vi "Update.vi"(10 "测试版？":bool, 11 "服务器信息":T1={"host"="27.154.58.30", "port"=8020, "user"="std", "password"="std23506", "远端地址"="/微站/室外总磷总氮高压过滤无主板新电路板/一体化微型水质监测站.exe"}) -> ()   [LabVIEW 2016, in "数据传输系统-03.lvlib" / "update.lvlib"]
uses:
  update.lvlib
  <vilib>/Utility/miscctls.llb/LVPointTypeDef.ctl
panel:
  out "引用输出":refnum<vi>
  out "已下载大小":sgl format="%.2f MB"
  out "滑动杆":dbl(slide) scale=0.0..100.0
  in  "取消按钮":bool
  out "last status string":string caption="最近状态字符串"
  out "command":string caption="命令"
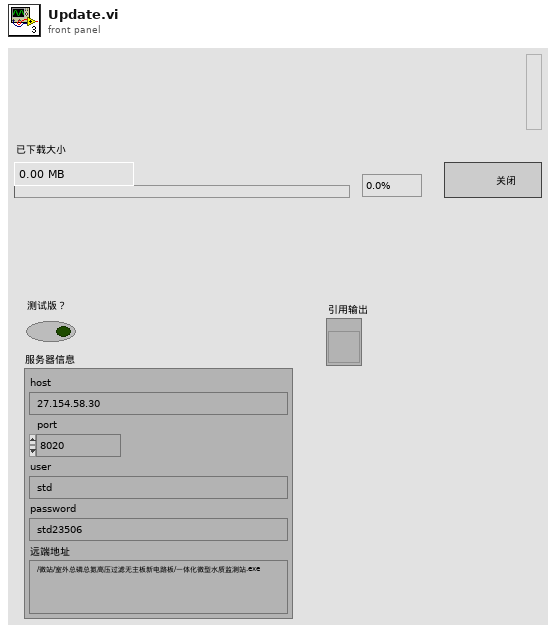
[diagram p1: front panel]
types:
  T1 = cluster{"host":string, "port":u16, "user":string, "password":string, "远端地址":string}
  T2 = typedef "LVPointTypeDef.ctl" = cluster{"Horizontal":i16, "Vertical":i16}
  T3 = cluster{"command":string, "last status string":string, "process":dbl}
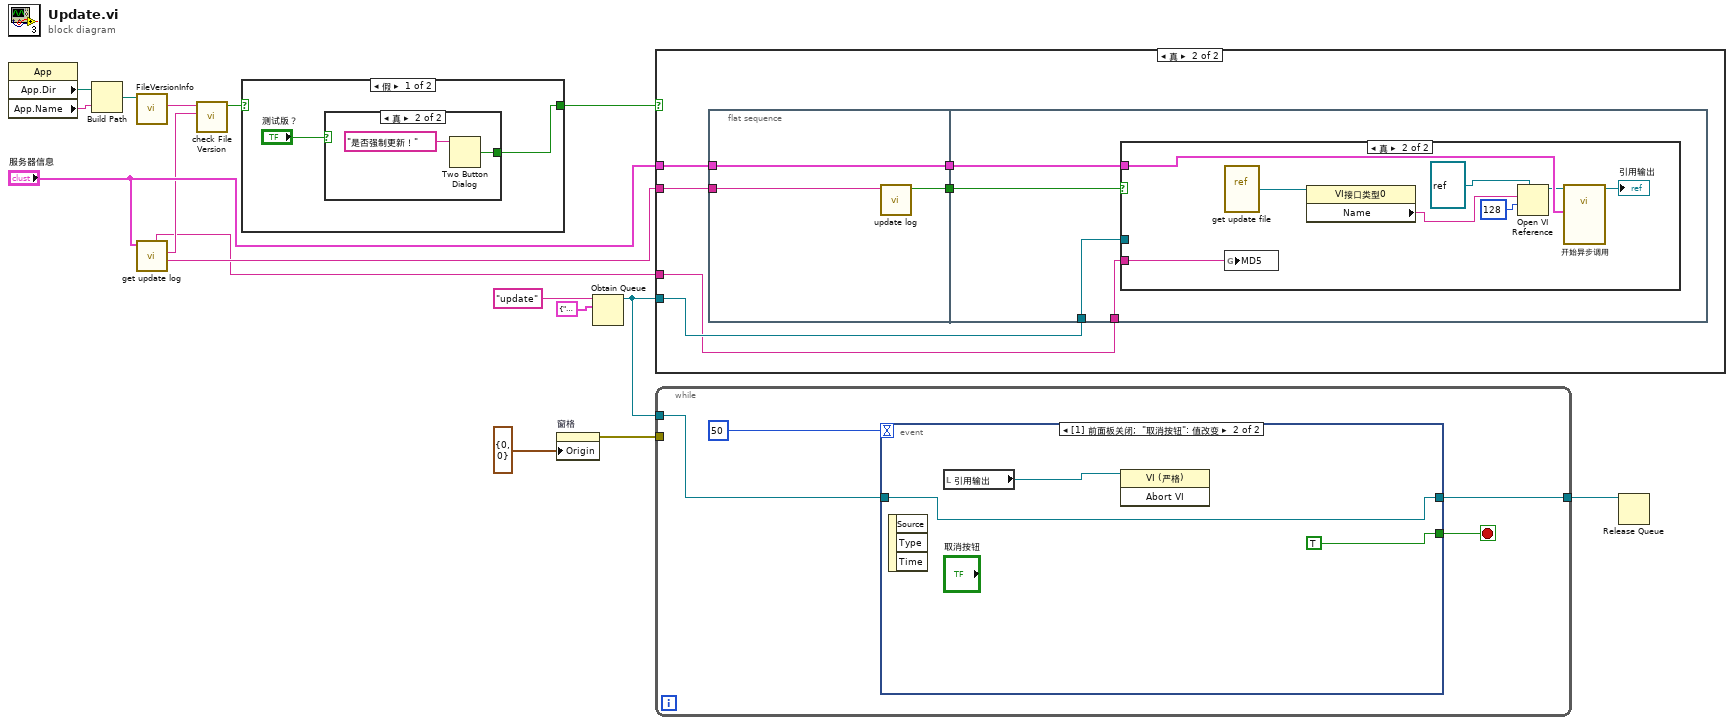
[diagram p0: block diagram]
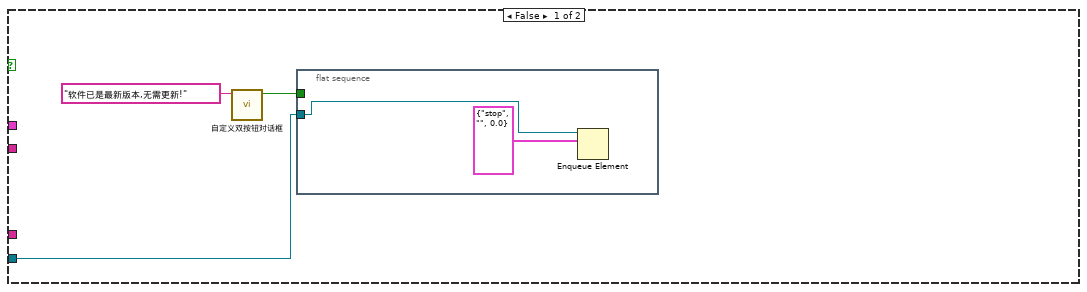
[diagram p4: hidden frame]
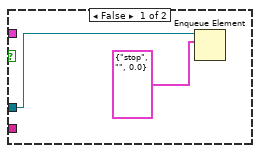
[diagram p5: hidden frame]
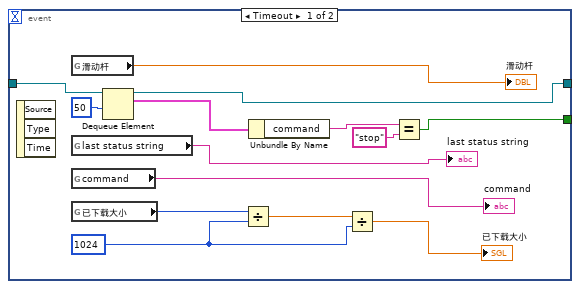
[diagram p6: hidden frame]
diagram:
  n1 = property class="App"() -> ("App.Dir"=w11:path, "App.Name"=w10:string)  [unwired: 2 in, 2 out]
  n2 = Build Path(base path=w11, name or relative path=w10) -> (appended path=w9:path)
  n3 = call <vilib>:"FileVersionInfo.vi"("Application Path in"=w9) -> ("File Version Info"=w6:string)  [unwired: 7 in, 3 out]
  n4 = call "get update log.vi"("服务器信息"="服务器信息") -> ("部分更新日志"=w7:string, "remote File Version"=w12:string, "MD5"=w5:string)  [unwired: 6 in, 2 out]
  n5 = call "check File Version.vi"("remote File Version Info"=w12, "Local File Version Info"=w6) -> ("new?"=w4:bool)  [unwired: 9 in]
  n6 = case shown="假" w4 {
    selector: w4 -> [_ w21]
    tunnel: [w17 w21] -> w3
    frame False {
      n7 = case shown="真" "测试版？" {
        tunnel: [_ w20] -> w17
        frame False {
        }
        frame True {
          n8 = Two Button Dialog(message="是否强制更新！" ("消息")) -> (T button?=w20:bool)  [unwired: 2 in]
        }
      }
    }
    frame True {
    }
  }
  n9 = property on="窗格" class="Pane"("Origin"=T2 {"Horizontal"=0, "Vertical"=0} ("原点")) -> (error out=w2:errorcluster)  [unwired: 2 in, 1 out]
  n10 = Obtain Queue(name (unnamed)="update" ("名称（未命名）"), element data type=T3 {"command"="", "last status string"="", "process"=0.0}) -> (queue out=w8:refnum<queue>)  [unwired: 3 in, 2 out]
  n11 = case shown="真" w3 {
    tunnel: "服务器信息" -> [_ w32]
    tunnel: w7 -> [_ w30]
    tunnel: w8 -> [w24 w28]
    tunnel: w5 -> [_ w27]
    frame False {
      n12 = call "自定义双按钮对话框.vi"("消息"="软件已是最新版本,无需更新!") -> ("输出"=w22:bool)  [unwired: 10 in]
      n13 = flat-sequence {
        tunnel: w24 -> [w26]
        tunnel: w22 -> [_]
        frame #0 {
          n14 = Enqueue Element(queue=w26, element=T3 {"command"="stop", "last status string"="", "process"=0.0} ("元素")) -> ()  [unwired: 2 in, 3 out]
        }
      }
    }
    frame True {
      n15 = flat-sequence {
        tunnel: w32 -> [w35]
        tunnel: [w35] -> w31
        tunnel: w30 -> [w34]
        tunnel: [w33] -> w29
        tunnel: w31 -> [w39]
        tunnel: w29 -> [w38]
        tunnel: w28 -> [w37]
        tunnel: w27 -> [w36]
        frame #0 {
          n16 = call "update log.vi"("更新记录"=w34) -> ("check"=w33:bool)  [unwired: 10 in]
        }
        frame #1 {
          n17 = case shown="真" w38 {
            tunnel: w39 -> [_ w47]
            tunnel: w37 -> [w40 _]
            tunnel: w36 -> [_ w46]
            frame False {
              n18 = Enqueue Element(queue=w40, element=T3 {"command"="stop", "last status string"="", "process"=0.0} ("元素")) -> ()  [unwired: 2 in, 3 out]
            }
            frame True {
              n19 = vi-ref "get update file.vi"() -> (w49:refnum<vi>)
              n20 = global write "更新全局变量.vi" "MD5"(w46) -> ()
              n21 = property class="VI接口类型0"(reference=w49) -> ("Name"=w48:string)  [unwired: 1 in, 2 out]
              n22 = Open VI Reference(type specifier VI Refnum (for type only)=refnum<vi> refnum, vi path=w48, options=128 ("选项")) -> (vi reference=w44:refnum<vi>)  [unwired: 3 in, 1 out]
              n23 = call-by-ref "开始异步调用"(reference=w44, "服务器信息"=w47) -> (reference out=→"引用输出":refnum<vi>)  [unwired: 12 in, 1 out]
            }
          }
        }
      }
    }
  }
  n24 = while {
    tunnel: w8 -> [w51]
    tunnel: [w50] -> w15
    tunnel: w2 -> [_]
    stop <- w52 stop-if-true
    n25 = event shown="[1] 前面板关闭;  \"取消按钮\": 值改变" {
      selector: _ -> [_ _]
      dyn-events: _ -> [_ _]
      timeout: 50 -> [_ _]
      tunnel: [w62 TRUE] -> w52
      tunnel: w51 -> [w67 w69]
      tunnel: [w65 w69] -> w50
      event Timeout {
        w55 = i64 1024 ("y")
        n26 = event-data() -> ()  [unwired: 1 in, 3 out]
        n27 = global read "更新全局变量.vi" "滑动杆"() -> (→"滑动杆":dbl)
        n28 = global read "更新全局变量.vi" "last status string"() -> (→"last status string":string)
        n29 = global read "更新全局变量.vi" "command"() -> (→"command":string)
        n30 = global read "更新全局变量.vi" "已下载大小"() -> (w57:i64)
        n31 = Dequeue Element(queue=w67, timeout in ms (-1)=50 ("超时毫秒(-1)")) -> (queue out=w65:refnum<queue>, element=w66:T3)  [unwired: 1 in, 2 out]
        n32 = Divide(x=w57, y=w55) -> (x/y=w56:dbl)
        n33 = Unbundle By Name(w66) -> ("command"=w64:string)
        n34 = Divide(x=w56, y=w55) -> (x/y=→"已下载大小":dbl)
        n35 = Equal?(x=w64, y="stop") -> (x = y?=w62:bool)
      }
      event Panel Close; "取消按钮": Value Change {
        n36 = event-data() -> ()  [unwired: 1 in, 3 out]
        n37 = local read "引用输出"() -> (w68:refnum<vi>)
        n38 = invoke class="VI (严格)" method="Abort VI"(reference=w68) -> ()  [unwired: 2 in, 3 out]
      }
    }
  }
  n39 = Release Queue(queue=w15) -> ()  [unwired: 2 in, 3 out]
